vi "readSPEHeader.vi"() -> ()   [LabVIEW 2015]
panel:
  out "int":i16
  out "short":i8
  out "long 2":i32
  out "long":i32
  out "float":sgl
  out "エラー出力":errorcluster
  in  "エラー入力":errorcluster
  out "exp_sec":sgl
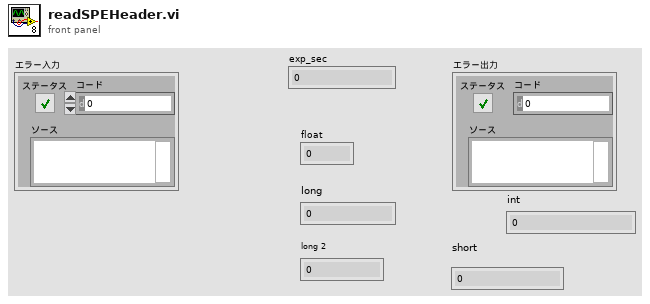
[diagram p1: front panel]
types:
  T1 = enum16{"open", "open or create", "create or replace", "create", "open (read only)"}
  T2 = enum16{"open", "replace", "create", "open or create", "replace or create", "replace or create with confirmation"}
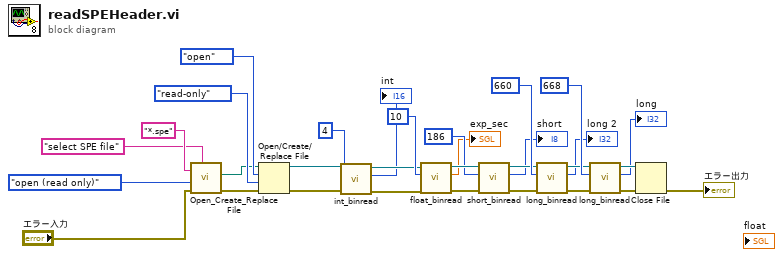
[diagram p0: block diagram]
diagram:
  n1 = call <vilib>:"Open_Create_Replace File.vi"("pattern"="*.spe", "prompt"="select SPE file", "error in (no error)"="エラー入力", "function (open:0)"=T1."open (read only)") -> ("error out"=w27:errorcluster, "new file path"=w28:path)  [unwired: 4 in, 2 out]
  n2 = Open/Create/Replace File(file path (use dialog)=w28, error in=w27, operation (0:open)=T2."open", access (0:read/write)=enum16{"read/write", "read-only", "write-only"}."read-only" ("アクセス （0:read/write）")) -> (refnum out=w6:refnum<file>, error out=w3:errorcluster)  [unwired: 2 in, 1 out]
  n3 = call "int_binread.vi"("error in"=w3, "offset"=i64 4, "ref in"=w6) -> ("error out"=w4:errorcluster, "int"=→"int":i16, "ref out"=w5:refnum<file>)  [unwired: 6 in]
  n4 = call "float_binread.vi"("error in"=w4, "offset"=i64 10, "ref in"=w5) -> ("error out"=w13:errorcluster, "float"=→"exp_sec":sgl, "ref out"=w12:refnum<file>)  [unwired: 6 in]
  n5 = call "short_binread.vi"("error in"=w13, "offset"=i64 186, "ref in"=w12) -> ("error out"=w20:errorcluster, "short"=→"short":i8, "ref out"=w21:refnum<file>)  [unwired: 6 in]
  n6 = call "long_binread.vi"("error in"=w20, "offset"=i64 660, "ref in"=w21) -> ("error out"=w19:errorcluster, "long"=→"long 2":i32, "ref out"=w15:refnum<file>)  [unwired: 6 in]
  n7 = call "long_binread.vi"("error in"=w19, "offset"=i64 668, "ref in"=w15) -> ("error out"=w18:errorcluster, "long"=→"long":i32, "ref out"=w17:refnum<file>)  [unwired: 6 in]
  n8 = Close File(refnum=w17, error in=w18) -> (error out=→"エラー出力":errorcluster)  [unwired: 1 out]
